vi "Bresenhams Line Algorithm LabVIEW 2012 NIVerified.vi"(9 "End":cluster{"X":i32, "Y":i32}, 11 "Start":cluster{"X":i32, "Y":i32}) -> (1 "Pixels":i32, 3 "Line Points":cluster{"X":i32, "Y":i32}[](array[cluster]))   [LabVIEW 2019]
doc: "Implementation of Bresenhams Line Algorithm in LabVIEW. This calculates the pixels that fall on a particular line.\nFrom pseudocode (with minor error fixed) from http://en.wikipedia.org/wiki/Bresenham%27s_line_algorithm \n\n function line(x0, y0, x1, y1)\n real deltax := x1 - x0\n real deltay := y1 - y0\n real deltaerr := abs(deltay / deltax) // Assume deltax != 0 (line is not vertical),\n // note that this division needs to be done in a way that preserves the fractional part\n real error := 0.0 // No error at start\n int y := y0\n for x from x0 to x1 \n plot(x,y)\n error := error + deltaerr\n if error = 0.5 then\n y := y + 1\n error := error - 1.0"
panel:
  # "Overview: Bresenham's Line Algorithm calculates the pixels on a line from a given start and end.\nRequirements: NI LabVIEW Base Development System 2012 (or compatible).\nInstructions: \n1. Write the Start and End coordinates.\n2. Run the VI."
  # "Based upon pseudo-code at http://en.wikipedia.org/wiki/Bresenham%27s_line_algorithm"
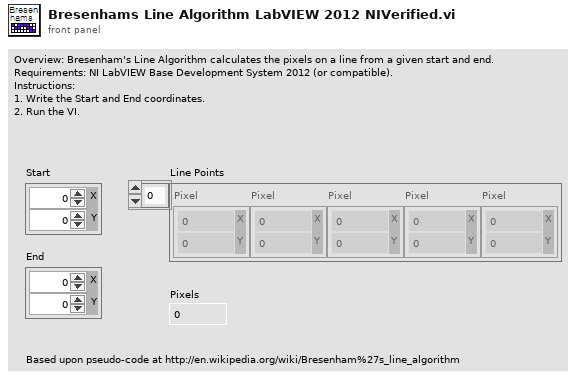
[diagram p1: front panel]
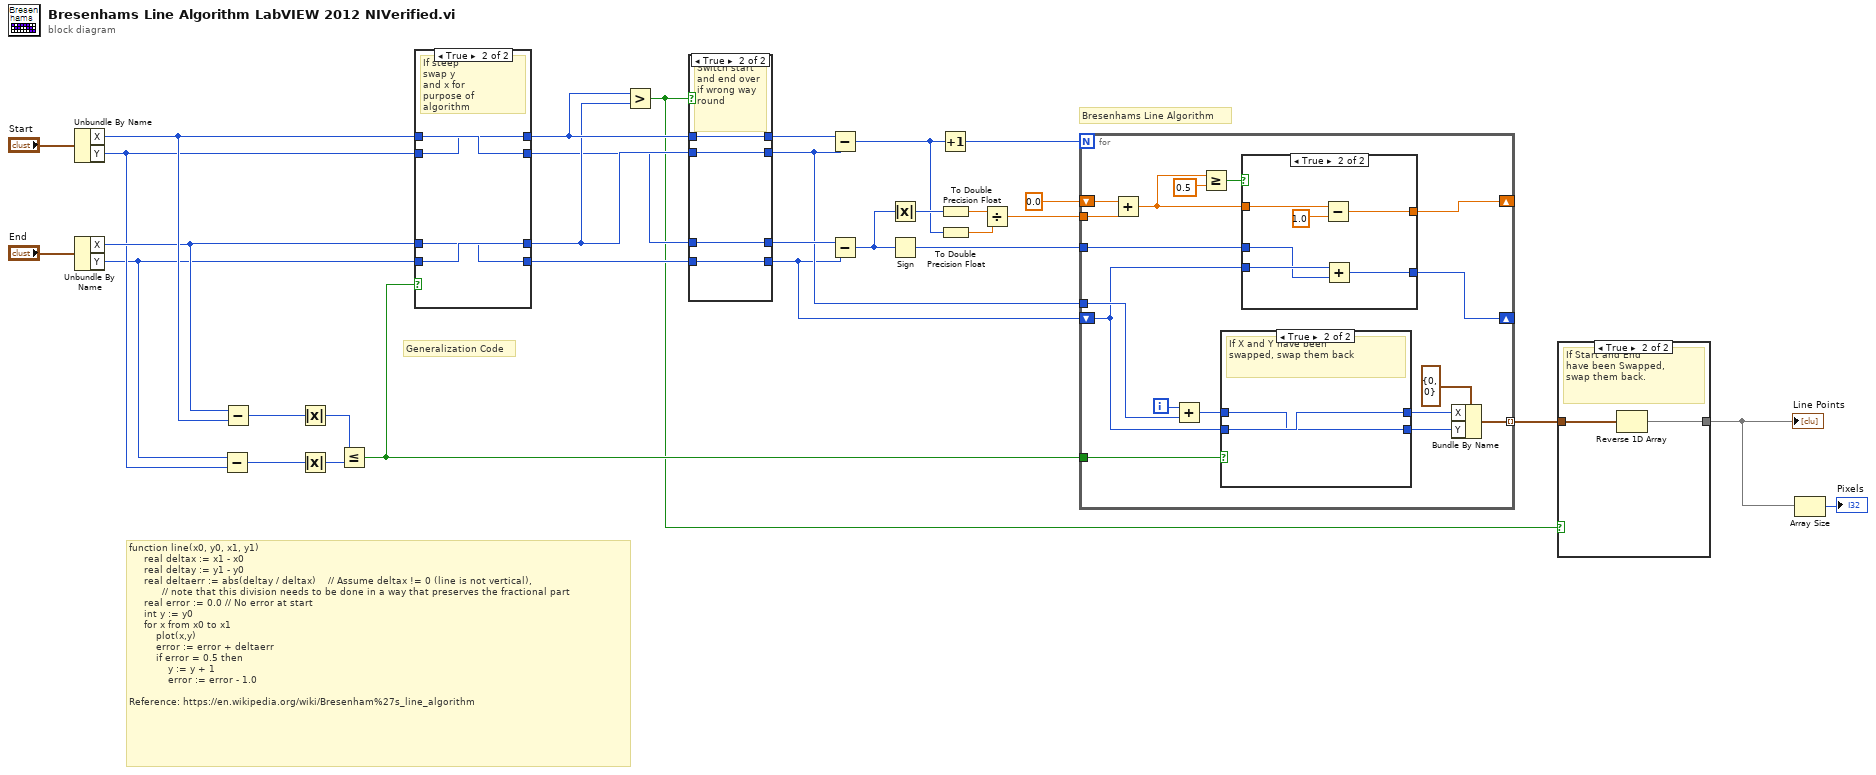
[diagram p0: block diagram]
diagram:
  # "function line(x0, y0, x1, y1)\n     real deltax := x1 - x0\n     real deltay := y1 - y0\n     real deltaerr := abs(deltay / deltax)    // Assume deltax != 0 (line is not vertical),\n           // note that this division needs to be done in a way that preserves the fractional part\n     real error := 0.0 // No error at start\n     int y := y0\n     for x from x0 to x1 \n         plot(x,y)\n         error := error + deltaerr\n         if error = 0.5 then\n             y := y + 1\n             error := error - 1.0\n\nReference: https://en.wikipedia.org/wiki/Bresenham%27s_line_algorithm"
  # "Bresenhams Line Algorithm"
  # "Generalization Code"
  n1 = Unbundle By Name("Start") -> ("X"=w26:i32, "Y"=w24:i32)
  n2 = Unbundle By Name("End") -> ("X"=w25:i32, "Y"=w23:i32)
  n3 = Subtract(x=w23, y=w24) -> (x-y=w29:i32)
  n4 = Subtract(x=w25, y=w26) -> (x-y=w30:i32)
  n5 = Absolute Value(x=w30) -> (abs(x)=w27:i32)
  n6 = Absolute Value(x=w29) -> (abs(x)=w28:i32)
  n7 = Less Or Equal?(x=w27, y=w28) -> (x <= y?=w9:bool)
  n8 = case shown="True" w9 {
    tunnel: w26 -> [w36 w40]
    tunnel: w25 -> [w35 w37]
    tunnel: w24 -> [w34 w39]
    tunnel: w23 -> [w33 w38]
    tunnel: [w34 w40] -> w20
    tunnel: [w33 w37] -> w19
    tunnel: [w36 w39] -> w22
    tunnel: [w35 w38] -> w21
    frame False {
    }
    frame True {
      # "If steep\nswap y\nand x for\npurpose of\nalgorithm"
    }
  }
  n9 = Greater?(x=w22, y=w21) -> (0:w6:bool)
  n10 = case shown="True" w6 {
    tunnel: w22 -> [w44 w48]
    tunnel: w21 -> [w43 w47]
    tunnel: w20 -> [w42 w46]
    tunnel: w19 -> [w41 w45]
    tunnel: [w44 w47] -> w14
    tunnel: [w43 w48] -> w18
    tunnel: [w42 w45] -> w11
    tunnel: [w41 w46] -> w17
    frame False {
    }
    frame True {
      # "Switch start\nand end over\nif wrong way\nround"
    }
  }
  n11 = Subtract(x=w18, y=w14) -> (x-y=w8:i32)
  n12 = Subtract(x=w17, y=w11) -> (x-y=w15:i32)
  n13 = Absolute Value(x=w15) -> (abs(x)=w16:i32)
  n14 = Sign(1:w15) -> (0:w10:i32)
  n15 = Increment(x=w8) -> (x+1=w7:i32)
  n16 = To Double Precision Float(number=w16) -> (double precision float=w3:dbl)
  n17 = To Double Precision Float(number=w8) -> (double precision float=w4:dbl)
  n18 = Divide(x=w3, y=w4) -> (x/y=w12:dbl)
  n19 = for {
    N: w7 -> [_]
    tunnel: w14 -> [w64]
    shift-right: [w51] -> _
    shift-left: 0.0 -> [w52]
    tunnel: w12 -> [w63]
    tunnel: w10 -> [w54]
    tunnel: w9 -> [w61]
    tunnel: [w57] -> w5 mode=indexing
    shift-right: [w53] -> _
    shift-left: w11 -> [w49]
    i -> [w65]
    n20 = Add(x=w52, y=w63) -> (x+y=w50:dbl)
    n21 = Add(x=w65, y=w64) -> (x+y=w59:i32)
    n22 = Greater Or Equal?(x=w50, y=0.5) -> (x >= y?=w56:bool)
    n23 = case shown="True" w61 {
      tunnel: w49 -> [w74 w77]
      tunnel: [w75 w77] -> w60
      tunnel: w59 -> [w75 w76]
      tunnel: [w74 w76] -> w58
      frame False {
      }
      frame True {
        # "If X and Y have been\nswapped, swap them back"
      }
    }
    n24 = case shown="True" w56 {
      tunnel: w49 -> [w66 w73]
      tunnel: w54 -> [_ w70]
      tunnel: [w66 w72] -> w53
      tunnel: w50 -> [w67 w71]
      tunnel: [w67 w69] -> w51
      frame False {
      }
      frame True {
        n25 = Subtract(x=w71, y=1.0) -> (x-y=w69:dbl)
        n26 = Add(x=w73, y=w70) -> (x+y=w72:i32)
      }
    }
    n27 = Bundle By Name(cluster=cluster{"X":i32, "Y":i32} {"X"=0, "Y"=0} ("Start"), "X"=w60, "Y"=w58) -> (w57:cluster{"X":i32, "Y":i32})
  }
  n28 = case shown="True" w6 {
    tunnel: w5 -> [w78 w80]
    tunnel: [w78 w79] -> w2
    frame False {
    }
    frame True {
      # "If Start and End\nhave been Swapped,\nswap them back."
      n29 = Reverse 1D Array(array=w80) -> (reversed array=w79:cluster{"X":i32, "Y":i32}[])
    }
  }
  "Line Points" <- w2
  n30 = Array Size(array=w2) -> (size(s)=→"Pixels":i32)
